vi "DB Tools Fetch Next Recordset.vi"   [LabVIEW 2012, in "NI_Database_API_64.lvlib"]
doc: "Retrieves the next recordset in a multi-recordset query identified by <B>recordset reference</B>. When the current recordset is no longer available, the <B>recordset reference</B> is redirected to the new recordset. Wire data to the reference input to determine the polymorphic instance to use or manually select the instance."
uses:
  NI_Database_API_64.lvlib
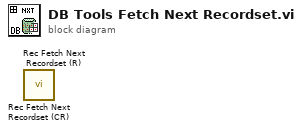
[diagram p0: block diagram]
diagram:
  n1 = call "Rec Fetch Next Recordset (CR).vi"() -> ()  [unwired: 6 in, 2 out]
  n2 = call "Rec Fetch Next Recordset (R).vi"() -> ()  [unwired: 6 in, 2 out]
